vi "Initialize Core.vi"(8 "error in":errorcluster, 10 "Shared Resources":refnum<class "Shared Resources.lvclass">, 11 "Logging Execution Unit in":refnum<class "Logging Execution Unit.lvclass">) -> (0 "error out":errorcluster, 3 "Logging Execution Unit out":refnum<class "Logging Execution Unit.lvclass">)   [LabVIEW 2020, in "AIM ARINC 429 Engine.lvlib" / "Implementation.lvlib" / "Logging Execution Unit.lvclass"]
uses:
  Logging Execution Unit.lvclass
  Hardware API/AIM ARINC 429 Hardware API.lvlib
  Logging/Word Logging/Word Logging.lvlib
  Logging/Word Logging/Log Producer/Log Producer.lvclass
  Shared Resources/Shared Resources.lvclass
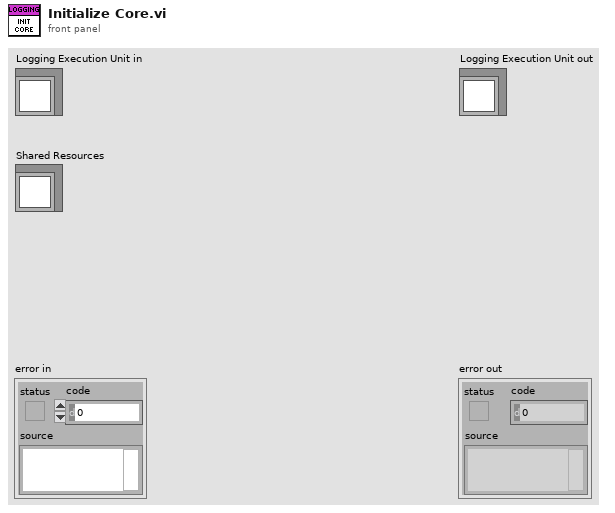
[diagram p1: front panel]
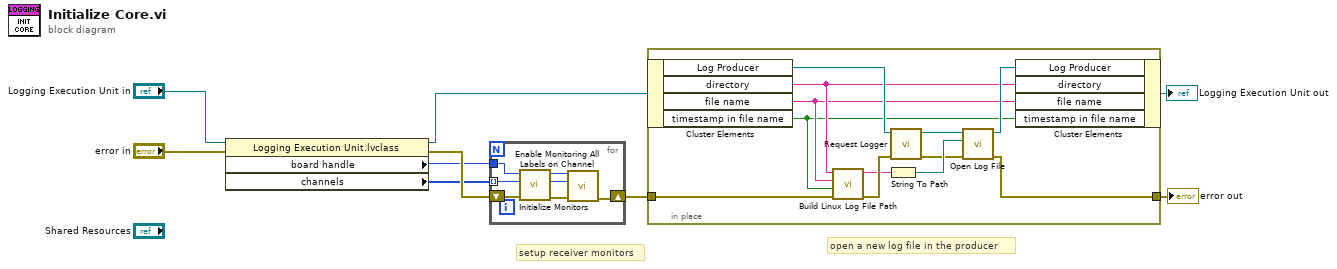
[diagram p0: block diagram]
diagram:
  # "open a new log file in the producer"
  # "setup receiver monitors"
  n1 = property class="Logging Execution Unit.lvclass"(reference="Logging Execution Unit in", error in="error in") -> (reference out=w4:refnum<class "Logging Execution Unit.lvclass">, error out=w9:errorcluster, "board handle"=w8:u8, "channels"=w6:u8[])
  n2 = for {
    tunnel: w6 -> [w11] mode=indexing
    shift-right: [w14] -> w3
    shift-left: w9 -> [w16]
    tunnel: w8 -> [w13]
    n3 = call "Initialize Monitors.vi"("error in"=w16, "channel number"=w11, "board handle"=w13) -> ("error out"=w15:errorcluster, "channel number out"=w10:u8, "board handle out"=w12:u8)  [unwired: 6 in]
    n4 = call "Enable Monitoring All Labels on Channel.vi"("error in"=w15, "channel number"=w10, "board handle"=w12) -> ("error out"=w14:errorcluster)  [unwired: 6 in, 2 out]
  }
  n5 = in-place {
    in-place-border: w3 -> [w27]
    in-place-border: [w22] -> w1
    n6 = in-place-cluster #1(w4) -> ("Log Producer"=w25:refnum<class "Log Producer.lvclass">, "directory"=w19:string, "file name"=w18:string, "timestamp in file name"=w17:bool)
    n7 = call "Build Linux Log File Path.vi"("error in (no error)"=w27, "Timestamp"=w17, "Name"=w18, "Log File Directory"=w19) -> ("error out"=w21:errorcluster, "Log File Path"=w20:string)  [unwired: 6 in]
    n8 = String To Path(string=w20) -> (path=w26:path)
    n9 = call "Request Logger.vi"("error in (no error)"=w21, "Producer in"=w25) -> ("error out"=w23:errorcluster, "Producer out"=w28:refnum<class "Log Producer.lvclass">)  [unwired: 8 in]
    n10 = call "Open Log File.vi"("error in (no error)"=w23, "Path"=w26, "Log Producer in"=w28) -> ("error out"=w22:errorcluster, "Log Producer out"=w24:refnum<class "Log Producer.lvclass">)  [unwired: 7 in]
    n11 = in-place-cluster #1("Log Producer"=w24, "directory"=w19, "file name"=w18, "timestamp in file name"=w17) -> (→"Logging Execution Unit out":refnum<class "Logging Execution Unit.lvclass">)
  }
  "error out" <- w1
